vi "Mutex Attr Init.vi"(8 "error in (no error)":errorcluster, 11 "Mutex Attr in":T1) -> (0 "error out":errorcluster, 3 "Mutex Attr out":T1)   [LabVIEW 2013, in "Linux RT IPC.lvlib" / "POSIX Threads.lvlib" / "Mutex Attr.lvclass"]
doc: "Calls pthread_mutexattr_init() on the pthread mutex attribute object encapsulated by Mutex Attr.\n\nThis VI initializes the mutex attribute object and sets its default values.\n\nRefer to online POSIX documentation for more information."
uses:
  Mutex Attr.lvclass
  Controls/reference.ctl
  POSIX Thread Object/POSIX Thread Object.lvclass/POSIX Thread Object.ctl
  POSIX Thread Object/Private VIs/libpthread path.vi
  POSIX Thread Object/Private VIs/get pthread error.vi
  POSIX Thread Object/POSIX Thread Object.lvclass
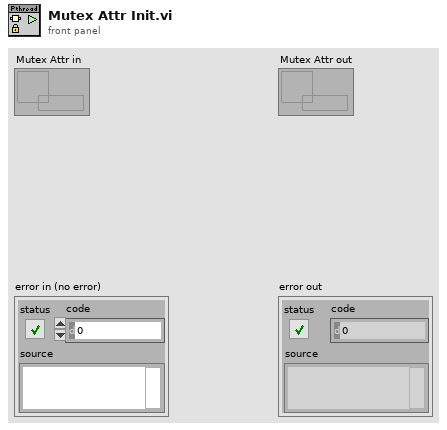
[diagram p1: front panel]
types:
  T1 = typedef "Linux RT IPC.lvlib/POSIX Threads.lvlib/Mutex Attr.lvclass/reference.ctl" = refnum<data-value>
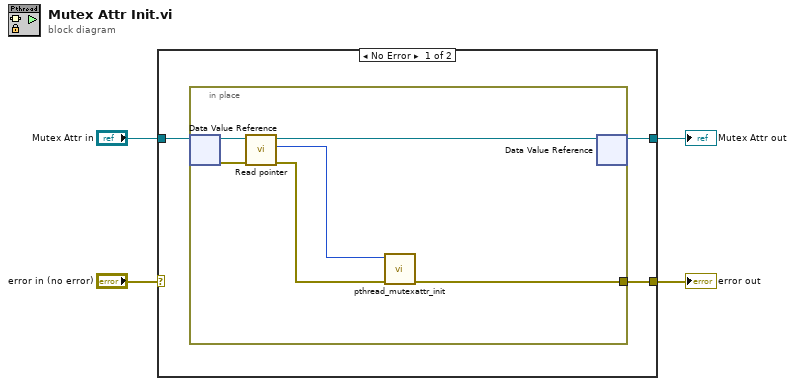
[diagram p0: block diagram]
diagram:
  n1 = case shown="No Error" "error in (no error)" {
    selector: "error in (no error)" -> [_ w15]
    tunnel: [w5 w15] -> w4
    tunnel: "Mutex Attr in" -> [w7 w14]
    tunnel: [w6 w14] -> w3
    frame No Error {
      n2 = in-place {
        in-place-border: [w9] -> w5
        n3 = in-place-dvr #1(w7) -> (w13:refnum<class "Mutex Attr.lvclass">, w11:errorcluster)
        n4 = call "Read pointer.vi"("error in (no error)"=w11, "POSIX Thread Object in"=w13) -> ("error out"=w10:errorcluster, "pointer"=w8:u64, "POSIX Thread Object out"=w12:refnum<class "Mutex Attr.lvclass">)  [unwired: 7 in]
        n5 = call "pthread_mutexattr_init.vi"("error in (no error)"=w10, "mutex attr ptr in"=w8) -> ("error out"=w9:errorcluster)  [unwired: 8 in, 1 out]
        n6 = in-place-dvr #1(w12) -> (w6:T1)  [unwired: 1 out]
      }
    }
    frame Error {
    }
  }
  "Mutex Attr out" <- w3
  "error out" <- w4
